vi "Write visible.vi"(8 "error in (no error)":errorcluster, 10 "visible":bool, 11 "TextDecoration in":refnum<class "TextDecoration.lvclass">) -> (0 "error out":errorcluster, 3 "TextDecoration out":refnum<class "TextDecoration.lvclass">)   [LabVIEW 2023, in "TLC_Scripto.lvlib" / "TextDecoration.lvclass"]
uses:
  TextDecoration.lvclass
  TextDecoration.lvclass/TextDecoration.ctl
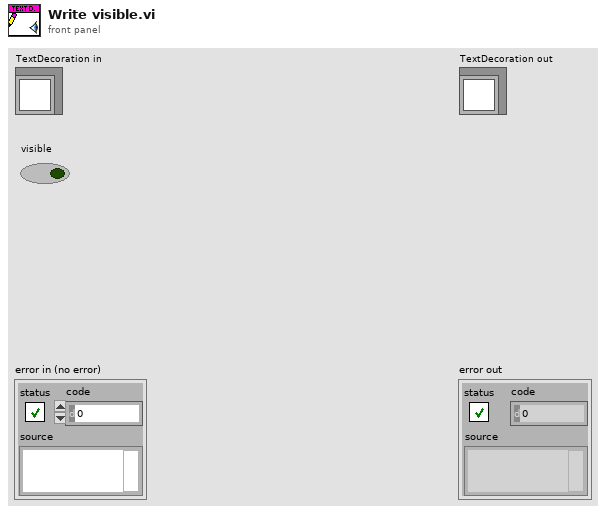
[diagram p1: front panel]
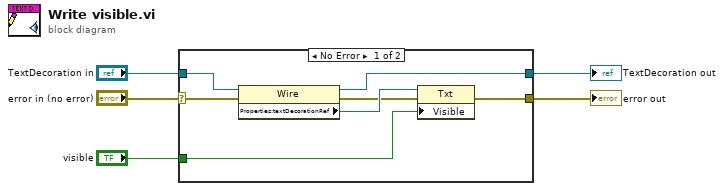
[diagram p0: block diagram]
diagram:
  n1 = case shown="No Error" "error in (no error)" {
    selector: "error in (no error)" -> [w7 w13]
    tunnel: [w6 w13] -> w4
    tunnel: [w9 w14] -> w2
    tunnel: "TextDecoration in" -> [w10 w14]
    tunnel: "visible" -> [w8 _]
    frame No Error {
      n2 = property class="Wire"(reference=w10, error in=w7) -> (reference out=w9:refnum<class "TextDecoration.lvclass">, error out=w11:errorcluster, "Properties:textDecorationRef"=w12:refnum<vi>)
      n3 = property class="Txt"(reference=w12, error in=w11, "Visible"=w8) -> (error out=w6:errorcluster)  [unwired: 1 out]
    }
    frame Error {
    }
  }
  "error out" <- w4
  "TextDecoration out" <- w2
